vi "Initialize.vi"(7 "timeout, ms (2000)":u32=2000, 8 "error in (no error)":errorcluster, 10 "product id (0x89B6)":u16=35254 format="%04x", 11 "vendor id (0x04D8)":u16=1240 format="%04x") -> (0 "error out":errorcluster, 3 "TroSpec out":refnum<class "PL ISTEQ TroSpec.lvclass">)   [LabVIEW 2015, in "PL ISTEQ TroSpec.lvclass"]
doc: "Initializes connection to device using specified settings."
uses:
  PL ISTEQ TroSpec.lvclass
  PL ISTEQ TroSpec.lvclass/PL ISTEQ TroSpec.ctl
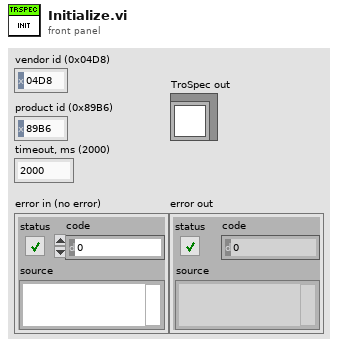
[diagram p1: front panel]
types:
  T1 = enum32{"invalid CPU target", "Motorola 68K", "PowerPC", "Intel x86", "SPARC", "PA-RISC", "MIPS", "Alpha", "ARM", "AMD/Intel x64"}
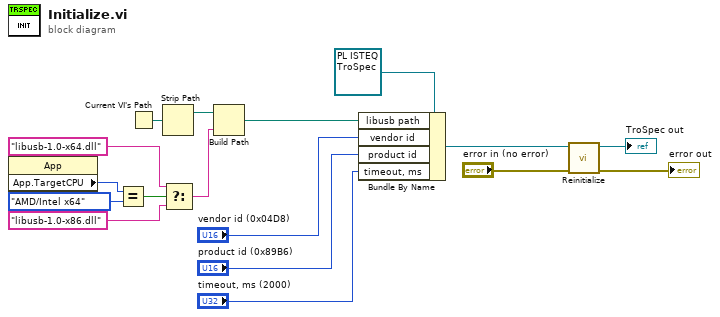
[diagram p0: block diagram]
diagram:
  n1 = property class="App"() -> ("App.TargetCPU"=w17:T1)  [unwired: 2 in, 2 out]
  n2 = Equal?(x=w17, y=T1."AMD/Intel x64" ("Application:Target:CPU")) -> (x = y?=w15:bool)
  n3 = Current VI's Path() -> (path=w14:path)
  n4 = Strip Path(path=w14) -> (stripped path=w13:path)  [unwired: 1 out]
  n5 = Select(t="libusb-1.0-x64.dll", s=w15, f="libusb-1.0-x86.dll") -> (s? t:f=w10:string)
  n6 = Build Path(base path=w13, name or relative path=w10) -> (appended path=w8:path)
  n7 = Bundle By Name(cluster=refnum<class "PL ISTEQ TroSpec.lvclass"> refnum ("Eltochpribor RRG.lvclass"), "libusb path"=w8, "vendor id"="vendor id (0x04D8)", "product id"="product id (0x89B6)", "timeout, ms"="timeout, ms (2000)") -> (w5:refnum<class "PL ISTEQ TroSpec.lvclass">)
  n8 = call "Reinitialize.vi"("error in (no error)"="error in (no error)", "TroSpec in"=w5) -> ("error out"=→"error out":errorcluster, "TroSpec out"=→"TroSpec out":refnum<class "PL ISTEQ TroSpec.lvclass">)  [unwired: 8 in]
